vi "Read address.vi"(8 "error in (no error)":errorcluster, 11 "WebsocketsConnection in":refnum<class "WebsocketsConnection.lvclass">) -> (0 "error out":errorcluster, 2 "address":string="localhost", 3 "WebsocketsConnection out":refnum<class "WebsocketsConnection.lvclass">)   [LabVIEW 2013, in "MQTT_Websockets.lvlib" / "WebsocketsConnection.lvclass"]
uses:
  WebsocketsConnection.lvclass
  WebsocketsConnection.lvclass/WebsocketsConnection.ctl
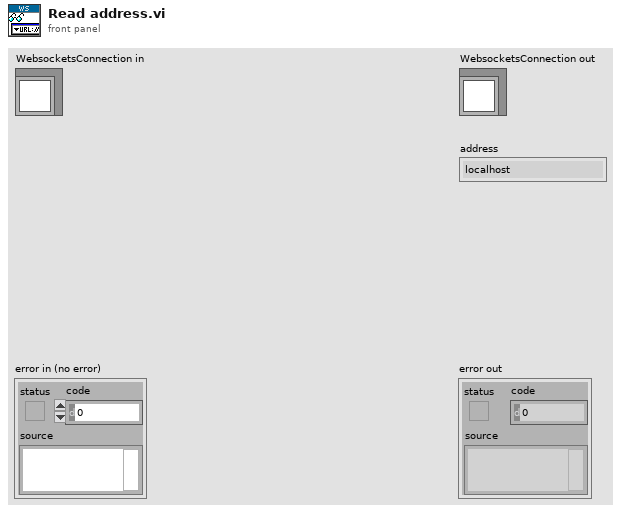
[diagram p1: front panel]
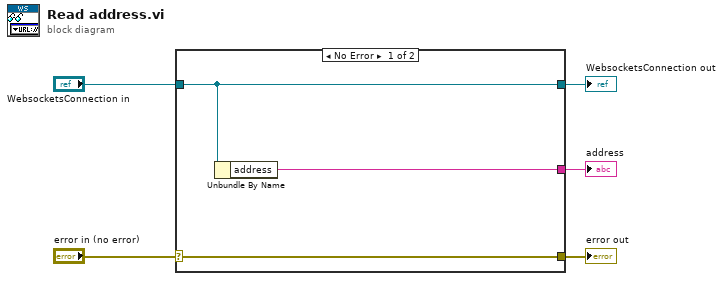
[diagram p0: block diagram]
diagram:
  n1 = case shown="No Error" "error in (no error)" {
    selector: "error in (no error)" -> [w8 w9]
    tunnel: [w8 w9] -> w4
    tunnel: [w7 w10] -> w2
    tunnel: "WebsocketsConnection in" -> [w7 w10]
    tunnel: [w6 _] -> w1
    frame No Error {
      n2 = Unbundle By Name(w7) -> ("address"=w6:string)
    }
    frame Error {
    }
  }
  "error out" <- w4
  "WebsocketsConnection out" <- w2
  "address" <- w1
